vi "niRFUtil RFHS FIFO Write.vi"(0 "Fifo ID":T2, 2 "Benchmark Task (Parent)":T1, 5 "IQ Samples":csg[](array[numeric]), 11 "error in (no error)":errorcluster) -> (4 "Fifo ID (out)":T2, 15 "error out":errorcluster)   [LabVIEW 2015, in "niRFUtil.lvlib"]
uses:
  niRFUtil.lvlib
  niRFUtil RFHS FIFO Reference.ctl
  niRFUtil RFHS FIFO.ctl
  Benchmark/niRFUtil RFHS Benchmark Task.ctl
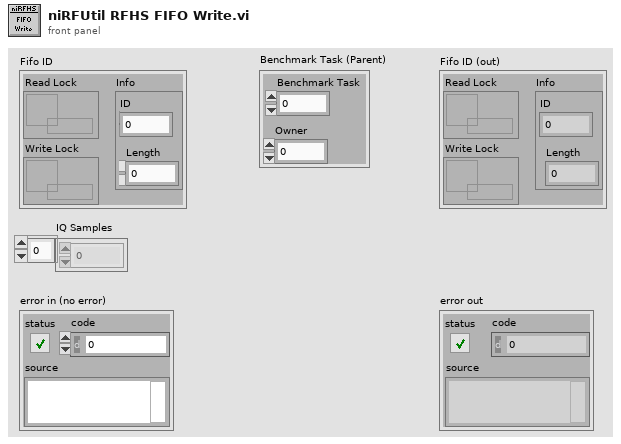
[diagram p1: front panel]
types:
  T1 = typedef "niRFUtil.lvlib/niRFUtil RFHS Benchmark Task.ctl" = cluster{"Benchmark Task":u64, "Owner":u32}
  T2 = typedef "niRFUtil.lvlib/niRFUtil RFHS FIFO Reference.ctl" = cluster{"Read Lock":refnum<data-value>, "Info":T3, "Write Lock":refnum<data-value>}
  T3 = typedef "niRFUtil.lvlib/niRFUtil RFHS FIFO.ctl" = cluster{"ID":u64, "Length":u32}
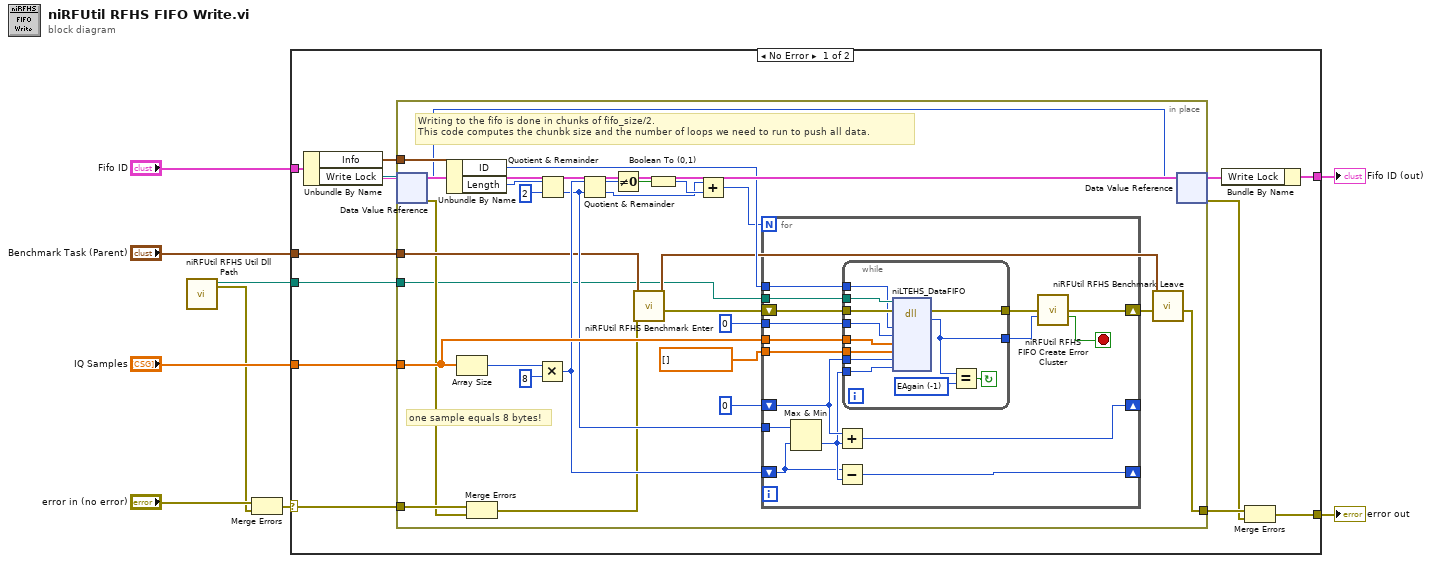
[diagram p0: block diagram]
diagram:
  n1 = call "niRFUtil RFHS Util Dll Path.vi"() -> ("error out"=w1:errorcluster, "Path"=w4:path)  [unwired: 7 in, 3 out]
  n2 = Merge Errors("error in (no error)", w1) -> (w2:errorcluster)
  n3 = case shown="No Error" w2 {
    selector: w2 -> [w20 w78]
    tunnel: "IQ Samples" -> [w21 _]
    tunnel: [w12 w78] -> w8
    tunnel: "Fifo ID" -> [w17 w77]
    tunnel: [w15 w77] -> w6
    tunnel: "Benchmark Task (Parent)" -> [w14 _]
    tunnel: w4 -> [w10 _]
    frame No Error {
      n4 = Unbundle By Name(w17) -> ("Info"=w18:T3, "Write Lock"=w19:refnum<data-value>)
      n5 = in-place {
        in-place-border: [w28] -> w13
        in-place-border: w21 -> [w46]
        in-place-border: w20 -> [w25]
        in-place-border: w18 -> [w31]
        in-place-border: w14 -> [w29]
        in-place-border: w10 -> [w22]
        # "Writing to the fifo is done in chunks of fifo_size/2. \nThis code computes the chunbk size and the number of loops we need to run to push all data."
        # "one sample equals 8 bytes!"
        n6 = in-place-dvr #1(w19) -> (w30:i32, w23:errorcluster)
        n7 = Unbundle By Name(w31) -> ("ID"=w43:u64, "Length"=w33:u32)
        n8 = Array Size(array=w46) -> (size(s)=w45:i32)
        n9 = Merge Errors(w25, w23) -> (w24:errorcluster)
        n10 = Multiply(x=w45, y=8) -> (x*y=w41:i32)
        n11 = Quotient & Remainder(x=w33, y=u32 2) -> (floor(x/y)=w32:u32)  [unwired: 1 out]
        n12 = Quotient & Remainder(x=w41, y=w32) -> (x-y*floor(x/y)=w40:u32, floor(x/y)=w37:u32)
        n13 = Not Equal To 0?(x=w40) -> (x != 0?=w39:bool)
        n14 = call "niRFUtil RFHS Benchmark Enter.vi"("error in (no error)"=w24, "Benchmark Task (Parent)"=w29) -> ("error out"=w26:errorcluster, "Benchmark Task (Self)"=w27:T1)  [unwired: 8 in]
        n15 = Boolean To (0,1)(Boolean=w39) -> (0, 1=w38:i16)
        n16 = Add(x=w37, y=w38) -> (x+y=w36:u32)
        n17 = for {
          N: w36 -> [_]
          tunnel: w22 -> [w64]
          tunnel: csg[] [] ("IQ Samples") -> [w63]
          tunnel: w46 -> [w62]
          tunnel: u32 0 ("what") -> [w60]
          tunnel: w43 -> [w59]
          shift-right: [w56] -> _
          shift-left: u32 0 -> [w58]
          shift-right: [w53] -> _
          shift-left: w41 -> [w54]
          tunnel: w32 -> [w57]
          shift-right: [w51] -> w48
          shift-left: w26 -> [w61]
          stop <- w49 stop-if-true
          n18 = Max & Min(x=w57, y=w54) -> (min(x,y)=w55:u32)  [unwired: 1 out]
          n19 = Add(x=w58, y=w55) -> (x+y=w56:u32)
          n20 = Subtract(x=w54, y=w55) -> (x-y=w53:u32)
          n21 = while {
            tunnel: w64 -> [w76]
            tunnel: [w75] -> w52
            tunnel: w63 -> [w74]
            tunnel: w62 -> [w73]
            tunnel: w55 -> [w72]
            tunnel: w61 -> [w71]
            tunnel: w60 -> [w70]
            tunnel: w59 -> [w69]
            tunnel: w58 -> [w67]
            tunnel: [w65] -> w50
            stop <- w68 continue-if-true
            w66 = -1 items=["OK"=1, "EAgain"=-1, "EZombie"=-2] ("Fifo error states")
            n22 = dll-call lib="M:/RfProtocols/RFmx/DLLs/niRFHS/trunk/2.0/dist/win32U/niRFHS_generic.dll" fn="niLTEHS_DataFIFO"(path in=w76, error in=w71, "fifoID"=w69, "what"=w70, "iBuf"=w73, "oBuf"=w74, "offset"=w67, "bytes"=w72) -> (error out=w75:errorcluster, "return type"=w65:i32)  [unwired: 7 in, 1 out]
            n23 = Equal?(x=w65, y=w66) -> (x = y?=w68:bool)
          }
          n24 = call "niRFUtil RFHS FIFO Create Error Cluster.vi"("error in (no error)"=w52, "fifo return value"=w50) -> ("error  out"=w51:errorcluster, "is error?"=w49:bool)  [unwired: 12 in]
        }
        n25 = call "niRFUtil RFHS Benchmark Leave.vi"("error in (no error)"=w48, "Benchmark Task Self"=w27) -> ("error out"=w28:errorcluster)  [unwired: 8 in, 1 out]
        n26 = in-place-dvr #1 ("Data Value Reference Read / Write Element")(w30) -> (w16:refnum<data-value>, w11:errorcluster)
      }
      n27 = Bundle By Name(cluster=w17, "Write Lock"=w16) -> (w15:T2)
      n28 = Merge Errors(w13, w11) -> (w12:errorcluster)
    }
    frame Error {
    }
  }
  "error out" <- w8
  "Fifo ID (out)" <- w6
